vi "countrate_viewer_pix25.vi"() -> ()   [LabVIEW 2022 SP3]
panel:
  in  "Current":u16(ring)=10 items=["010_0417_101816", "020_0417_101556", "040_0417_101120", "060_0417_100851", "080_0417_100615", "100_0417_100344", "120_0417_100115", "140_0417_095846", "160_0417_095605", "180_0417_095308", "200_0417_095036"]
  in  "Path":path=path "C:/Users/User/OneDrive/measurements/pix25/PIX25/17_04_2023/M1/1_CountRate_gate_1s_iKRUM_14_setting_1/TS_step_10"
  in  "Tab Control":enum32{"Single pixel", "Pixels ROI"}(tab)=enum."Pixels ROI"
  out "Counns_vs_Current":cluster{i32[], i32[]}(graph)={[10, 20, 40, 60, 80, 100, 120, 140, 160, 180, 200], [1269, 2399, 4745, 7025, 8884, 10294, 11332, 12142, 12811, 11997, 8843]}
  out "SP_Thscans":i32[][](graph)=[[1, 1, 1, 1, 1, 1, 1, 1, 1, 1, 2, 2, 189750, 27421, 55263, 771071, 189820, 555977, 604477, 176470, 8254, 2553, 2142, 2098, 1983, 1841, 1720, 1662, 1491, 1416, 1364, 1330, 1269, 1152, 1093, 1054, 962, 959, 932, 842, 859, 771, 782, 672, 660, 595, 542, 499, 515, 482, 463, 399, 324, 318, 310, 306, 275, 226, 206, 204, 183, 191, 154, 133, 105, 88, 81, 74, 55, 30, 16, 16, 9, 2, 1, 1, 1, 2, 0, 1, 1, 1, 1, 0, 1, 1, 1, 0, 0, 0, 0, 0, 0, 0, 0, 0, 0, 0, 0, 0, 0], [1, 1, 1, 1, 1, 1, 1, 1, 3, 3, 3, 6, 215655, 123107, 60400, 109023, 562715, 135760, 344132, 161375, 9801, 4778, 4548, 4138, 3957, 3703, 3430, 3172, 3013, 2937, 2749, 2622, 2399, 2350, 2299, 2087, 1990, 1901, 1845, 1667, 1682, 1571, 1407, 1320, 1305, 1218, 1205, 1051, 948, 927, 902, 820, 705, 694, 632, 587, 520, 474, 459, 424, 399, 303, 295, 270, 214, 207, 180, 122, 113, 80, 39, 26, 10, 5, 3, 2, 3, 3, 2, 1, 0, 2, 3, 0, 0, 0, 1, 0, 1, 1, 2, 0, 0, 1, 0, 0, 0, 0, 0, 2, 0], [1, 1, 1, 1, 1, 1, 1, 1, 2, 2, 6, 9, 246177, 154316, 61581, 291268, 92235, 808784, 175375, 162478, 14536, 9814, 8979, 8241, 7781, 7331, 6713, 6502, 6202, 5729, 5414, 5293, 4745, 4666, 4367, 4187, 4099, 3805, 3617, 3379, 3236, 2941, 2924, 2720, 2530, 2322, 2186, 2120, 1914, 1753, 1680, 1555, 1433, 1277, 1214, 1119, 1051, 921, 872, 761, 735, 644, 567, 508, 460, 399, 349, 302, 233, 134, 89, 44, 27, 11, 9, 10, 7, 4, 0, 2, 2, 1, 1, 2, 1, 1, 0, 0, 1, 1, 0, 2, 1, 1, 0, 0, 0, 0, 0, 0, 1], [1, 1, 1, 1, 1, 1, 1, 1, 1, 5, 11, 17, 251777, 562574, 84697, 446485, 689648, 558243, 122437, 148538, 18881, 13957, 12791, 11866, 11229, 10474, 9746, 9238, 8754, 8227, 7810, 7238, 7025, 6523, 6383, 5947, 5555, 5367, 5101, 4876, 4580, 4293, 4092, 3850, 3612, 3351, 3193, 2949, 2792, 2702, 2356, 2236, 2030, 1884, 1737, 1644, 1413, 1411, 1239, 1123, 1113, 932, 832, 746, 629, 568, 503, 412, 288, 228, 116, 62, 33, 22, 14, 6, 9, 5, 7, 4, 4, 3, 2, 5, 1, 2, 2, 1, 3, 1, 1, 0, 0, 1, 0, 0, 1, 0, 0, 0, 0], [1, 1, 1, 1, 1, 1, 1, 1, 2, 7, 9, 9, 202033, 1022635, 119268, 1015096, 454383, 182206, 350774, 170408, 22775, 17422, 15771, 14821, 13787, 12976, 12251, 11478, 10931, 10429, 9679, 9276, 8884, 8347, 7999, 7558, 7315, 6797, 6383, 6210, 5707, 5417, 5063, 4826, 4510, 4230, 3969, 3814, 3585, 3213, 3062, 2900, 2662, 2346, 2209, 1943, 1827, 1688, 1550, 1395, 1307, 1150, 1078, 943, 825, 699, 585, 452, 322, 237, 131, 73, 46, 27, 20, 10, 9, 5, 7, 1, 7, 4, 5, 1, 3, 4, 3, 3, 4, 2, 0, 0, 0, 0, 1, 0, 0, 0, 0, 1, 0], [1, 1, 1, 1, 1, 1, 2, 1, 3, 4, 11, 19, 274433, 736852, 821692, 369364, 339077, 400614, 49867, 156608, 25953, 20145, 18691, 17666, 16423, 15179, 14099, 13351, 12750, 11986, 11698, 10689, 10294, 9752, 9185, 8633, 8319, 7879, 7376, 7210, 6582, 6262, 5932, 5747, 5351, 4921, 4701, 4447, 4104, 3904, 3562, 3318, 3035, 2758, 2556, 2267, 2131, 1940, 1864, 1662, 1461, 1371, 1197, 1084, 930, 806, 719, 580, 439, 277, 172, 95, 36, 26, 14, 12, 12, 10, 8, 10, 4, 1, 5, 7, 5, 2, 2, 1, 5, 1, 2, 1, 0, 1, 2, 0, 1, 0, 0, 0, 1], [1, 1, 1, 1, 1, 1, 1, 2, 4, 7, 10, 12, 311804, 152117, 828999, 642634, 363185, 305129, 867296, 125119, 26655, 22309, 20313, 19079, 17994, 16979, 15927, 14965, 14006, 13378, 12576, 11787, 11332, 10840, 10197, 9767, 9169, 8727, 8266, 7729, 7339, 7013, 6584, 6047, 5921, 5521, 5177, 4875, 4525, 4121, 4020, 3700, 3209, 3060, 2771, 2622, 2360, 2146, 1955, 1821, 1658, 1461, 1314, 1171, 1072, 904, 782, 621, 477, 336, 173, 103, 46, 37, 27, 10, 16, 6, 16, 9, 9, 5, 8, 7, 5, 1, 3, 3, 1, 3, 2, 2, 0, 2, 3, 2, 1, 3, 1, 1, 0], [1, 1, 1, 1, 1, 1, 1, 1, 1, 8, 8, 20, 366384, 586024, 65549, 888105, 959806, 722112, 664736, 126970, 28637, 23922, 22045, 20230, 19190, 18013, 16934, 15760, 15137, 14055, 13485, 12874, 12142, 11633, 10788, 10428, 9923, 9586, 8835, 8358, 7772, 7294, 7183, 6704, 6305, 5917, 5557, 5285, 4911, 4634, 4218, 3980, 3659, 3388, 3186, 2909, 2580, 2378, 2168, 1935, 1806, 1563, 1444, 1285, 1215, 926, 829, 712, 496, 357, 218, 114, 64, 29, 22, 25, 15, 11, 13, 10, 4, 10, 4, 5, 5, 6, 3, 4, 2, 2, 3, 1, 2, 1, 0, 1, 1, 0, 0, 1, 2], [1, 1, 1, 1, 1, 1, 1, 1, 2, 3, 5, 7, 308514, 175649, 361198, 671641, 1026371, 658278, 908428, 135148, 29294, 24322, 22324, 21165, 19477, 18508, 17428, 16326, 15558, 14629, 13820, 13092, 12811, 11864, 11317, 10598, 10203, 9338, 8959, 8586, 8105, 7835, 7134, 6915, 6558, 6290, 5900, 5457, 4961, 4629, 4282, 3990, 3592, 3468, 3141, 2925, 2728, 2386, 2175, 2023, 1855, 1666, 1539, 1284, 1165, 985, 878, 728, 553, 356, 229, 135, 78, 34, 33, 17, 16, 6, 8, 8, 4, 8, 6, 5, 10, 3, 2, 4, 6, 3, 2, 2, 1, 3, 1, 0, 0, 3, 0, 0, 0], [1, 1, 1, 1, 1, 1, 1, 1, 2, 2, 5, 11, 362041, 673975, 623187, 712352, 72767, 287790, 813455, 131860, 28336, 23579, 21491, 20346, 19052, 17661, 16587, 15674, 14749, 14122, 13390, 12559, 11997, 11243, 10817, 10425, 9366, 9242, 8585, 8354, 7747, 7409, 7150, 6494, 6059, 5904, 5530, 5039, 4786, 4402, 4174, 3906, 3672, 3341, 3065, 2840, 2530, 2366, 2156, 1953, 1762, 1622, 1492, 1271, 1165, 972, 858, 703, 510, 331, 214, 148, 69, 47, 22, 30, 15, 11, 12, 13, 10, 15, 6, 12, 5, 7, 1, 3, 4, 4, 1, 2, 1, 1, 3, 0, 0, 1, 0, 0, 0], [1, 1, 1, 1, 1, 1, 1, 1, 1, 2, 2, 9, 291425, 195362, 891949, 260720, 603938, 253434, 410135, 175520, 23257, 17183, 16078, 14754, 13718, 12922, 12197, 11578, 11092, 10303, 9717, 9350, 8843, 8441, 7803, 7662, 7122, 6707, 6354, 6082, 5631, 5399, 5193, 4886, 4424, 4377, 4047, 3830, 3535, 3386, 3095, 3018, 2727, 2562, 2307, 2125, 1961, 1757, 1703, 1477, 1338, 1287, 1168, 1072, 906, 794, 641, 532, 392, 294, 183, 101, 93, 49, 25, 24, 16, 15, 8, 13, 15, 11, 5, 12, 3, 4, 4, 6, 4, 3, 4, 1, 0, 1, 2, 3, 1, 1, 0, 1, 0]]
  out "ROI_Thscans":i32[][](graph)
  out "ROI Counns_vs_Current":cluster{"x":i32[], "y":i32[]}[](graph)=[{"x"=[10, 20, 40, 60, 80, 100, 120, 140, 160, 180, 200], "y"=[5788, 11550, 22908, 34725, 46596, 58476, 69984, 80642, 89685, 96090, 95086]}, {"x"=[10, 20, 40, 60, 80, 100, 120, 140, 160, 180, 200], "y"=[5229, 10481, 21003, 31934, 43040, 53953, 63920, 73197, 81464, 86557, 82444]}, {"x"=[10, 20, 40, 60, 80, 100, 120, 140, 160, 180, 200], "y"=[6347, 12619, 24813, 37516, 50152, 62999, 76048, 88087, 97906, 105623, 107728]}, {"x"=[10, 20, 40, 60, 80, 100, 120, 140, 160, 180, 200], "y"=[5885, 12506, 24598, 33614, 44225, 60163, 71358, 71080, 88038, 99015, 103830]}, {"x"=[10, 20, 40, 60, 80, 100, 120, 140, 160, 180, 200], "y"=[7259, 14155, 27794, 42464, 55513, 68152, 83308, 97868, 111207, 117116, 122425]}, {"x"=[10, 20, 40, 60, 80, 100, 120, 140, 160, 180, 200], "y"=[6068, 11921, 24401, 36511, 48958, 61586, 73018, 85686, 98316, 100964, 106641]}, {"x"=[10, 20, 40, 60, 80, 100, 120, 140, 160, 180, 200], "y"=[5792, 11917, 25031, 37218, 50888, 63603, 76543, 90713, 98707, 107263, 103432]}, {"x"=[10, 20, 40, 60, 80, 100, 120, 140, 160, 180, 200], "y"=[5642, 11098, 21720, 33554, 45976, 58183, 67268, 77320, 84854, 93133, 85305]}, {"x"=[10, 20, 40, 60, 80, 100, 120, 140, 160, 180, 200], "y"=[4783, 9367, 19364, 30110, 40670, 52250, 61461, 68636, 71992, 73708, 66528]}, {"x"=[10, 20, 40, 60, 80, 100, 120, 140, 160, 180, 200], "y"=[6141, 12215, 23243, 35325, 46885, 54262, 66265, 74464, 84272, 95326, 103957]}, {"x"=[10, 20, 40, 60, 80, 100, 120, 140, 160, 180, 200], "y"=[6203, 12445, 23795, 36401, 47597, 60300, 71348, 83522, 92454, 105103, 105201]}, {"x"=[10, 20, 40, 60, 80, 100, 120, 140, 160, 180, 200], "y"=[6409, 12362, 24510, 36727, 48593, 60932, 73260, 84142, 99493, 104084, 102507]}, {"x"=[10, 20, 40, 60, 80, 100, 120, 140, 160, 180, 200], "y"=[5600, 10780, 21268, 32773, 44254, 56029, 68450, 78702, 89054, 95249, 91650]}, {"x"=[10, 20, 40, 60, 80, 100, 120, 140, 160, 180, 200], "y"=[5730, 11768, 23959, 37583, 51069, 65900, 77496, 87689, 90185, 88684, 82954]}, {"x"=[10, 20, 40, 60, 80, 100, 120, 140, 160, 180, 200], "y"=[4950, 9918, 20223, 31416, 43335, 51753, 63319, 71716, 76073, 80119, 73536]}, {"x"=[10, 20, 40, 60, 80, 100, 120, 140, 160, 180, 200], "y"=[5855, 11461, 22694, 33519, 44291, 54105, 63924, 75411, 84569, 90629, 94843]}, {"x"=[10, 20, 40, 60, 80, 100, 120, 140, 160, 180, 200], "y"=[7035, 13784, 26383, 39929, 53572, 64999, 77282, 92097, 103221, 112618, 117835]}, {"x"=[10, 20, 40, 60, 80, 100, 120, 140, 160, 180, 200], "y"=[5765, 11431, 22765, 34091, 46220, 56797, 69511, 81444, 89921, 98431, 97594]}, {"x"=[10, 20, 40, 60, 80, 100, 120, 140, 160, 180, 200], "y"=[5960, 11917, 23994, 36280, 49990, 62024, 74217, 91174, 99338, 105110, 100869]}, {"x"=[10, 20, 40, 60, 80, 100, 120, 140, 160, 180, 200], "y"=[5270, 10448, 20294, 32674, 44417, 56893, 68709, 77593, 86101, 90185, 82577]}, {"x"=[10, 20, 40, 60, 80, 100, 120, 140, 160, 180, 200], "y"=[5359, 10654, 22577, 35638, 47792, 61620, 74326, 84194, 92202, 95489, 86340]}, {"x"=[10, 20, 40, 60, 80, 100, 120, 140, 160, 180, 200], "y"=[6457, 12820, 25205, 37866, 48731, 60735, 70570, 80672, 88335, 98136, 114030]}, {"x"=[10, 20, 40, 60, 80, 100, 120, 140, 160, 180, 200], "y"=[5797, 11642, 22214, 32620, 43952, 52970, 65365, 76095, 85027, 94971, 99189]}, {"x"=[10, 20, 40, 60, 80, 100, 120, 140, 160, 180, 200], "y"=[6493, 13283, 25578, 38607, 51756, 65289, 78759, 90712, 102590, 112174, 113346]}, {"x"=[10, 20, 40, 60, 80, 100, 120, 140, 160, 180, 200], "y"=[6131, 12307, 23551, 36815, 47661, 62888, 75943, 87844, 97315, 101982, 101180]}, {"x"=[10, 20, 40, 60, 80, 100, 120, 140, 160, 180, 200], "y"=[5259, 10834, 21749, 33639, 45440, 57438, 67358, 78134, 85389, 90884, 82024]}, {"x"=[10, 20, 40, 60, 80, 100, 120, 140, 160, 180, 200], "y"=[5026, 10318, 21215, 32005, 44148, 54883, 64405, 72077, 78718, 81244, 72589]}, {"x"=[10, 20, 40, 60, 80, 100, 120, 140, 160, 180, 200], "y"=[5582, 11514, 22061, 33105, 43254, 53653, 62929, 72403, 81026, 90626, 100266]}, {"x"=[10, 20, 40, 60, 80, 100, 120, 140, 160, 180, 200], "y"=[6515, 13112, 25125, 38215, 50598, 59696, 72448, 86988, 92126, 106792, 112252]}, {"x"=[10, 20, 40, 60, 80, 100, 120, 140, 160, 180, 200], "y"=[5871, 11473, 22330, 34446, 46442, 59285, 70761, 83949, 95121, 101300, 100708]}, {"x"=[10, 20, 40, 60, 80, 100, 120, 140, 160, 180, 200], "y"=[5975, 11687, 23489, 38233, 51732, 64832, 78464, 90732, 100917, 108118, 99798]}, {"x"=[10, 20, 40, 60, 80, 100, 120, 140, 160, 180, 200], "y"=[6661, 13099, 26413, 39649, 53440, 67206, 82751, 93695, 99245, 104438, 102789]}, {"x"=[10, 20, 40, 60, 80, 100, 120, 140, 160, 180, 200], "y"=[4751, 9818, 20106, 31147, 42094, 53245, 62450, 70843, 77155, 77204, 68750]}, {"x"=[10, 20, 40, 60, 80, 100, 120, 140, 160, 180, 200], "y"=[5815, 11487, 23408, 33532, 43607, 53632, 62532, 72778, 91492, 87705, 93606]}, {"x"=[10, 20, 40, 60, 80, 100, 120, 140, 160, 180, 200], "y"=[6145, 12137, 24283, 35912, 47984, 60042, 71197, 82450, 91465, 101640, 106800]}, {"x"=[10, 20, 40, 60, 80, 100, 120, 140, 160, 180, 200], "y"=[5839, 12102, 23689, 34731, 47713, 58801, 72762, 84188, 95085, 103475, 101085]}, {"x"=[10, 20, 40, 60, 80, 100, 120, 140, 160, 180, 200], "y"=[6521, 13603, 26423, 40081, 53619, 67033, 81659, 94386, 102889, 112719, 101456]}, {"x"=[10, 20, 40, 60, 80, 100, 120, 140, 160, 180, 200], "y"=[5739, 11197, 23126, 35612, 47982, 62907, 73736, 83529, 91879, 97873, 91141]}, {"x"=[10, 20, 40, 60, 80, 100, 120, 140, 160, 180, 200], "y"=[4776, 10027, 20606, 32724, 45375, 55568, 68749, 77146, 85954, 87124, 78963]}, {"x"=[10, 20, 40, 60, 80, 100, 120, 140, 160, 180, 200], "y"=[6465, 12945, 25114, 37590, 48827, 59668, 70517, 82063, 86884, 102328, 112073]}, {"x"=[10, 20, 40, 60, 80, 100, 120, 140, 160, 180, 200], "y"=[6207, 12819, 24802, 36733, 48964, 60019, 73296, 82568, 95584, 103564, 111240]}, {"x"=[10, 20, 40, 60, 80, 100, 120, 140, 160, 180, 200], "y"=[6078, 11835, 23313, 35613, 48090, 59502, 70746, 83346, 92527, 100503, 98288]}, {"x"=[10, 20, 40, 60, 80, 100, 120, 140, 160, 180, 200], "y"=[6193, 12155, 24087, 37497, 49914, 62886, 79012, 89470, 101446, 105122, 106578]}, {"x"=[10, 20, 40, 60, 80, 100, 120, 140, 160, 180, 200], "y"=[5811, 11991, 23388, 36058, 48982, 61667, 73617, 84283, 93739, 96720, 89162]}, {"x"=[10, 20, 40, 60, 80, 100, 120, 140, 160, 180, 200], "y"=[4886, 9903, 19341, 30333, 40315, 52926, 62987, 71919, 76575, 80727, 72620]}, {"x"=[10, 20, 40, 60, 80, 100, 120, 140, 160, 180, 200], "y"=[5917, 11703, 22607, 32632, 44146, 54678, 61541, 69228, 77442, 83939, 88770]}, {"x"=[10, 20, 40, 60, 80, 100, 120, 140, 160, 180, 200], "y"=[6360, 12712, 25071, 37607, 49119, 61550, 73999, 87091, 99370, 110387, 117315]}, {"x"=[10, 20, 40, 60, 80, 100, 120, 140, 160, 180, 200], "y"=[5637, 10800, 21419, 31264, 42918, 52823, 63600, 74037, 85304, 92844, 92865]}, {"x"=[10, 20, 40, 60, 80, 100, 120, 140, 160, 180, 200], "y"=[6220, 12356, 24573, 37282, 46557, 62650, 77112, 90296, 96570, 105338, 98824]}, {"x"=[10, 20, 40, 60, 80, 100, 120, 140, 160, 180, 200], "y"=[5946, 11720, 22796, 34835, 47576, 61628, 74813, 81560, 88298, 94278, 89055]}, {"x"=[10, 20, 40, 60, 80, 100, 120, 140, 160, 180, 200], "y"=[4651, 9451, 20681, 30069, 45212, 52739, 60191, 77864, 84655, 86936, 76579]}, {"x"=[10, 20, 40, 60, 80, 100, 120, 140, 160, 180, 200], "y"=[5889, 11281, 22190, 31896, 40719, 51446, 59490, 68869, 78595, 86368, 91330]}, {"x"=[10, 20, 40, 60, 80, 100, 120, 140, 160, 180, 200], "y"=[6630, 12783, 24842, 37375, 48062, 59641, 71324, 81593, 90246, 97990, 104775]}, {"x"=[10, 20, 40, 60, 80, 100, 120, 140, 160, 180, 200], "y"=[5867, 11588, 22851, 33832, 47580, 60283, 70110, 82428, 96106, 103789, 98846]}, {"x"=[10, 20, 40, 60, 80, 100, 120, 140, 160, 180, 200], "y"=[6433, 13032, 25341, 39210, 52431, 65238, 82194, 94816, 104057, 110054, 109354]}, {"x"=[10, 20, 40, 60, 80, 100, 120, 140, 160, 180, 200], "y"=[4915, 9914, 21494, 33076, 44294, 56920, 67429, 73270, 86682, 91358, 86386]}, {"x"=[10, 20, 40, 60, 80, 100, 120, 140, 160, 180, 200], "y"=[4611, 9128, 18396, 29533, 42824, 55432, 65914, 75697, 77030, 74034, 65796]}, {"x"=[10, 20, 40, 60, 80, 100, 120, 140, 160, 180, 200], "y"=[6137, 12103, 24402, 35787, 46322, 56926, 68189, 78092, 88057, 96498, 103136]}, {"x"=[10, 20, 40, 60, 80, 100, 120, 140, 160, 180, 200], "y"=[5341, 10444, 20124, 29946, 40031, 49103, 59705, 69520, 78755, 87109, 92424]}, {"x"=[10, 20, 40, 60, 80, 100, 120, 140, 160, 180, 200], "y"=[6347, 12678, 25005, 37948, 50926, 63899, 77741, 91027, 102143, 113237, 111110]}, {"x"=[10, 20, 40, 60, 80, 100, 120, 140, 160, 180, 200], "y"=[5896, 11568, 23123, 35248, 47989, 60353, 71932, 85292, 93325, 98051, 96866]}, {"x"=[10, 20, 40, 60, 80, 100, 120, 140, 160, 180, 200], "y"=[5621, 11047, 21641, 34136, 46265, 58159, 71885, 81485, 90722, 94160, 87324]}, {"x"=[10, 20, 40, 60, 80, 100, 120, 140, 160, 180, 200], "y"=[4908, 10240, 20741, 31984, 42422, 54864, 64949, 74232, 78588, 79502, 74459]}, {"x"=[10, 20, 40, 60, 80, 100, 120, 140, 160, 180, 200], "y"=[5519, 11315, 22027, 32503, 44054, 53734, 63339, 68779, 79605, 90438, 94246]}, {"x"=[10, 20, 40, 60, 80, 100, 120, 140, 160, 180, 200], "y"=[5327, 10564, 20408, 30522, 40634, 50688, 60780, 70850, 82725, 89584, 94259]}, {"x"=[10, 20, 40, 60, 80, 100, 120, 140, 160, 180, 200], "y"=[5187, 10424, 20525, 31012, 41198, 52463, 61740, 72292, 80737, 88660, 92462]}, {"x"=[10, 20, 40, 60, 80, 100, 120, 140, 160, 180, 200], "y"=[6370, 12815, 25194, 38037, 52694, 66015, 80638, 94768, 104818, 109896, 103806]}, {"x"=[10, 20, 40, 60, 80, 100, 120, 140, 160, 180, 200], "y"=[5723, 10990, 22726, 34728, 45870, 62613, 72672, 81240, 94012, 98624, 94279]}, {"x"=[10, 20, 40, 60, 80, 100, 120, 140, 160, 180, 200], "y"=[5559, 11192, 22678, 35288, 48484, 61341, 72279, 82473, 89803, 91719, 83563]}, {"x"=[10, 20, 40, 60, 80, 100, 120, 140, 160, 180, 200], "y"=[6005, 12042, 23062, 34393, 44232, 53695, 63943, 74377, 83983, 92363, 99282]}, {"x"=[10, 20, 40, 60, 80, 100, 120, 140, 160, 180, 200], "y"=[5794, 11547, 22710, 33545, 44618, 55489, 66517, 76634, 86503, 95392, 101789]}, {"x"=[10, 20, 40, 60, 80, 100, 120, 140, 160, 180, 200], "y"=[5837, 11660, 22902, 33966, 46069, 58176, 70161, 82035, 93023, 101031, 102975]}, {"x"=[10, 20, 40, 60, 80, 100, 120, 140, 160, 180, 200], "y"=[6053, 11435, 23633, 35910, 47721, 60268, 72564, 83037, 92895, 99531, 95991]}, {"x"=[10, 20, 40, 60, 80, 100, 120, 140, 160, 180, 200], "y"=[6258, 12469, 24752, 38229, 51998, 64560, 79473, 91376, 97613, 104591, 96109]}, {"x"=[10, 20, 40, 60, 80, 100, 120, 140, 160, 180, 200], "y"=[4745, 9591, 19882, 31415, 42795, 54495, 64641, 72414, 77929, 80465, 74201]}, {"x"=[10, 20, 40, 60, 80, 100, 120, 140, 160, 180, 200], "y"=[5890, 11920, 23303, 34657, 45365, 55920, 65499, 75196, 82071, 93600, 101374]}, {"x"=[10, 20, 40, 60, 80, 100, 120, 140, 160, 180, 200], "y"=[6541, 12794, 25171, 36938, 48706, 60632, 71441, 88076, 93485, 103440, 108524]}, {"x"=[10, 20, 40, 60, 80, 100, 120, 140, 160, 180, 200], "y"=[5655, 11337, 22572, 34920, 46195, 57303, 68226, 77536, 91103, 95817, 102231]}, {"x"=[10, 20, 40, 60, 80, 100, 120, 140, 160, 180, 200], "y"=[6626, 13255, 26320, 40370, 54265, 67717, 82949, 96862, 107169, 113581, 108973]}, {"x"=[10, 20, 40, 60, 80, 100, 120, 140, 160, 180, 200], "y"=[5007, 10140, 19755, 29852, 40078, 51879, 61423, 71617, 79569, 84995, 75201]}, {"x"=[10, 20, 40, 60, 80, 100, 120, 140, 160, 180, 200], "y"=[5334, 10982, 21744, 34144, 47626, 59909, 72436, 82566, 84666, 86131, 77781]}, {"x"=[10, 20, 40, 60, 80, 100, 120, 140, 160, 180, 200], "y"=[6084, 12087, 23285, 34517, 44678, 55291, 64703, 74419, 83810, 94472, 100272]}, {"x"=[10, 20, 40, 60, 80, 100, 120, 140, 160, 180, 200], "y"=[5164, 10216, 19707, 29678, 38834, 48652, 58129, 66631, 75838, 84002, 91042]}, {"x"=[10, 20, 40, 60, 80, 100, 120, 140, 160, 180, 200], "y"=[5820, 11498, 22338, 33675, 45330, 56861, 67623, 79589, 87076, 93086, 95194]}, {"x"=[10, 20, 40, 60, 80, 100, 120, 140, 160, 180, 200], "y"=[5774, 11404, 23271, 36059, 47887, 61395, 73184, 84913, 95896, 103925, 99419]}, {"x"=[10, 20, 40, 60, 80, 100, 120, 140, 160, 180, 200], "y"=[5888, 11334, 22798, 34962, 47261, 60599, 72413, 82649, 93459, 96465, 87559]}, {"x"=[10, 20, 40, 60, 80, 100, 120, 140, 160, 180, 200], "y"=[5001, 10473, 21191, 32918, 45508, 57752, 67568, 75288, 84375, 85714, 80045]}, {"x"=[10, 20, 40, 60, 80, 100, 120, 140, 160, 180, 200], "y"=[5980, 11777, 23028, 34868, 46002, 56858, 65963, 76769, 85511, 94476, 103688]}, {"x"=[10, 20, 40, 60, 80, 100, 120, 140, 160, 180, 200], "y"=[6195, 12294, 23971, 34973, 46585, 58801, 69267, 80044, 91049, 100823, 105158]}, {"x"=[10, 20, 40, 60, 80, 100, 120, 140, 160, 180, 200], "y"=[5630, 11163, 21926, 32709, 43989, 55769, 66330, 76422, 88035, 95997, 94069]}, {"x"=[10, 20, 40, 60, 80, 100, 120, 140, 160, 180, 200], "y"=[5857, 11599, 23570, 35384, 47865, 60303, 74962, 84949, 94807, 101965, 103666]}, {"x"=[10, 20, 40, 60, 80, 100, 120, 140, 160, 180, 200], "y"=[5007, 10073, 19834, 30441, 41982, 52912, 63872, 74633, 81127, 84755, 79298]}, {"x"=[10, 20, 40, 60, 80, 100, 120, 140, 160, 180, 200], "y"=[5078, 10291, 20946, 32363, 44816, 56083, 67671, 77244, 84536, 87080, 68102]}]
  out "Image":i32[][](graph)
  in  "ThScan_Load":bool
  in  "Exit":bool
  # "counts vs. current for single pixel for single vt"
  # "thscans of all currents for single pixel"
  # "counts vs. current for ROI pixels for single vt"
  # "thscans of ROI pixels for single current"
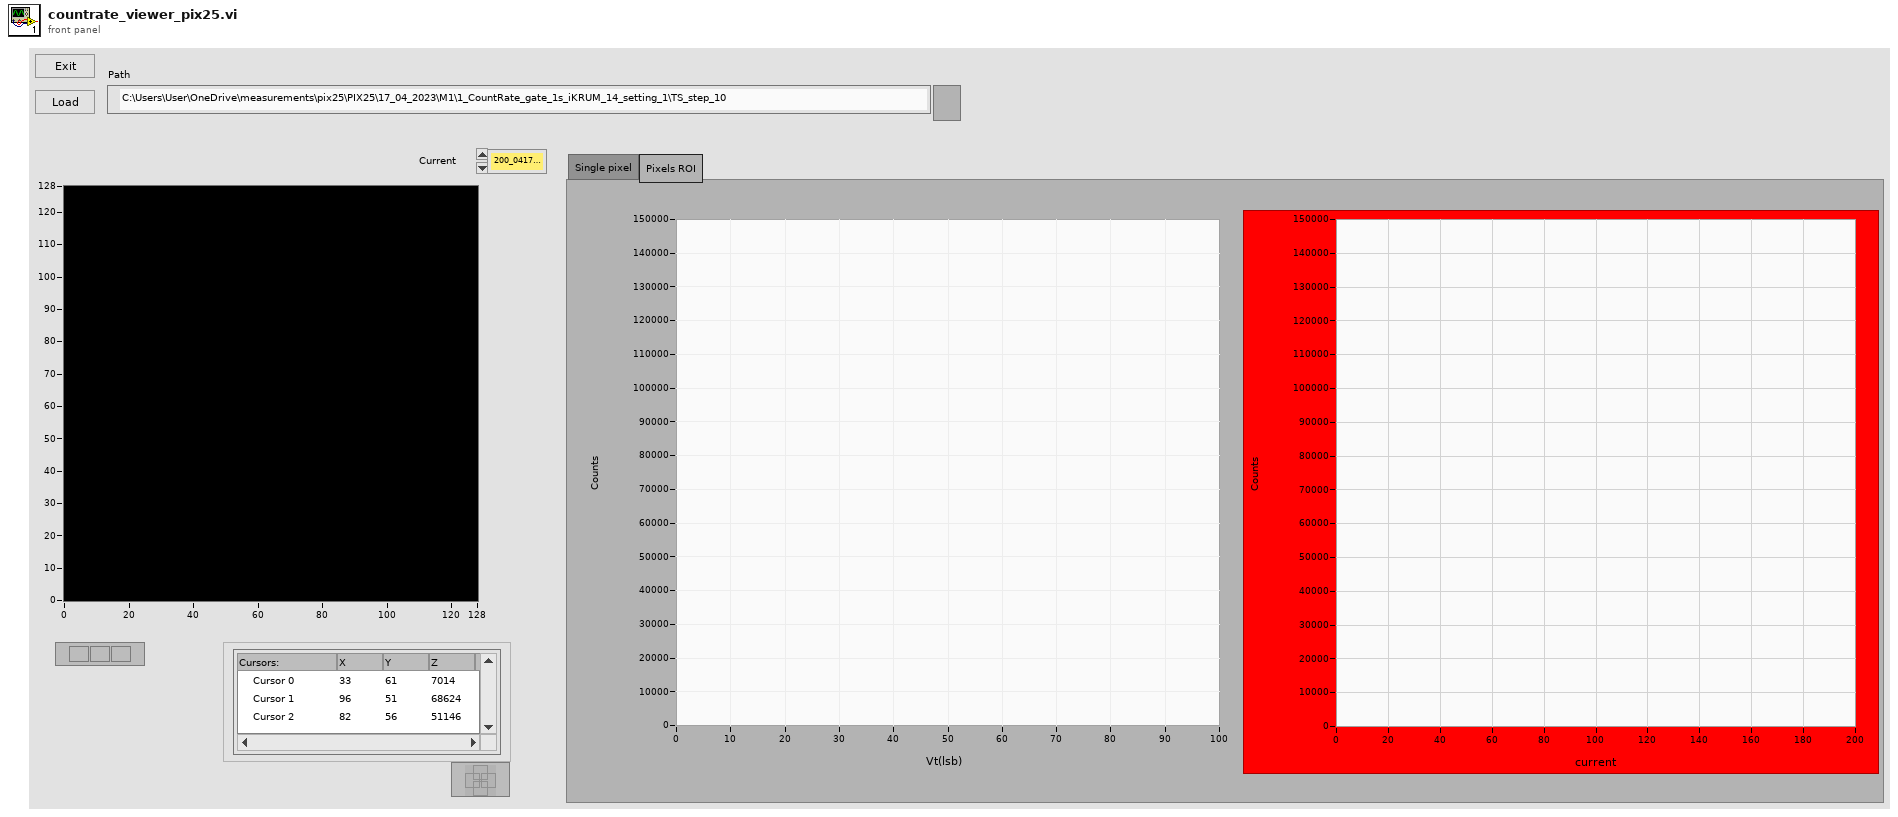
[diagram p1: front panel]
types:
  T1 = typedef "LVPointDoubleTypeDef.ctl" = cluster{"Cursor X":dbl, "Cursor Y":dbl}
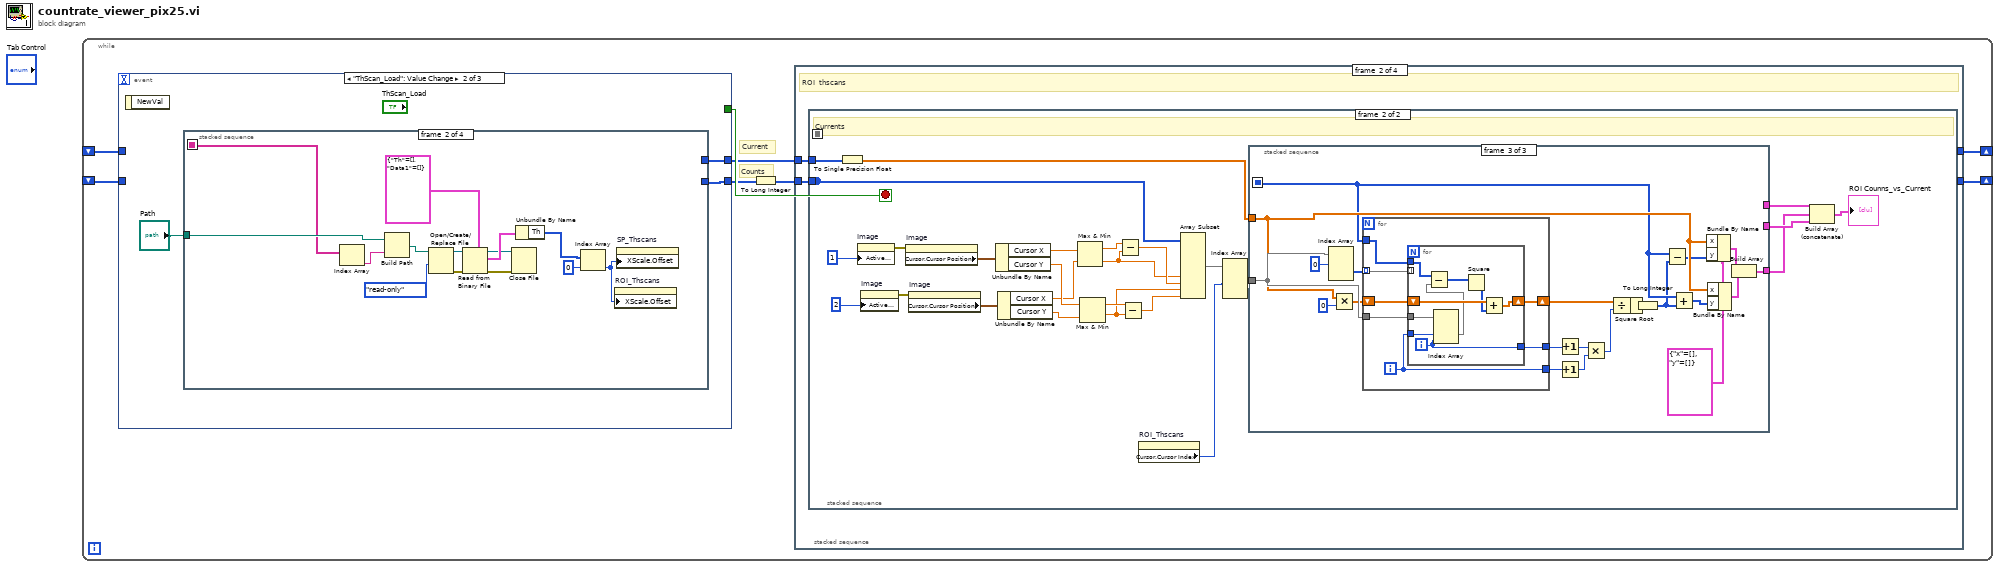
[diagram p0: block diagram]
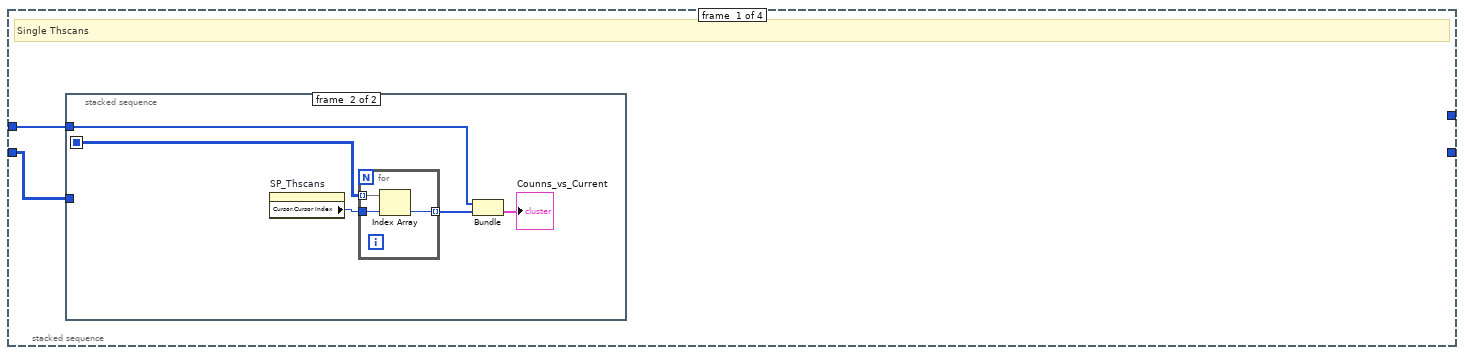
[diagram p2: hidden frame]
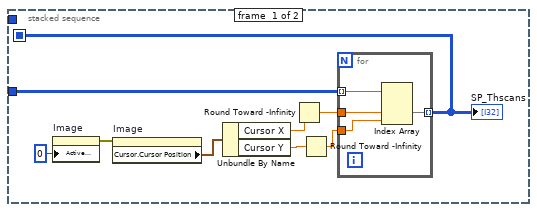
[diagram p3: hidden frame]
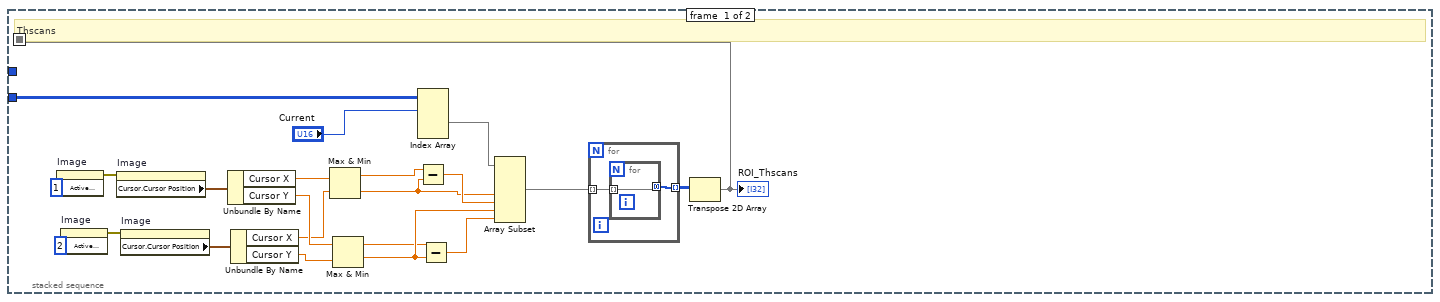
[diagram p4: hidden frame]
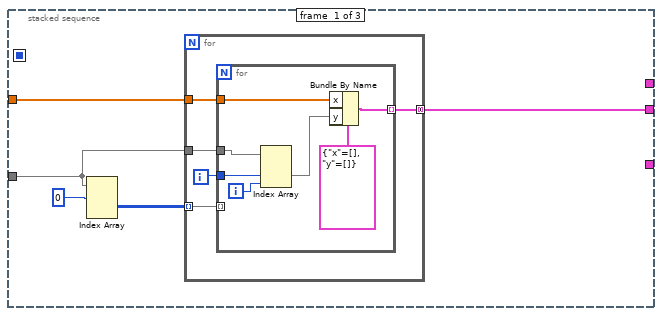
[diagram p5: hidden frame]
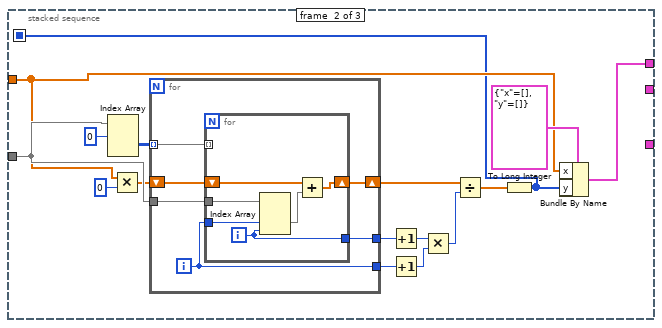
[diagram p6: hidden frame]
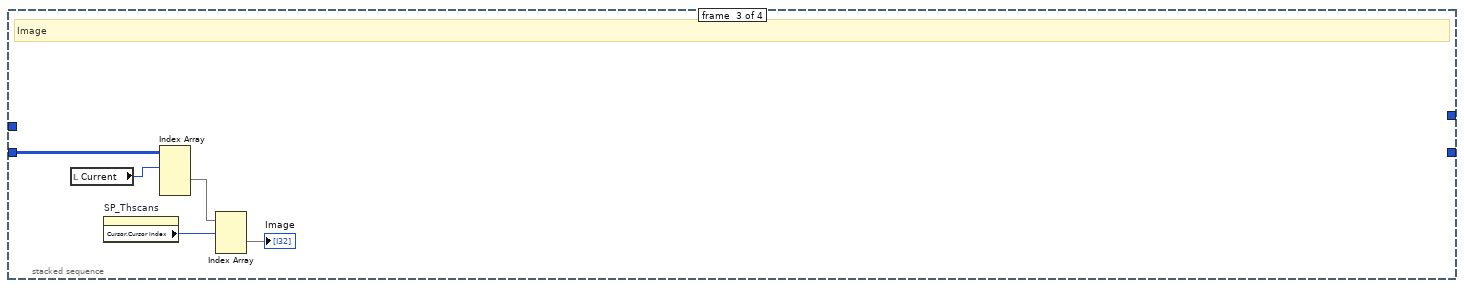
[diagram p7: hidden frame]
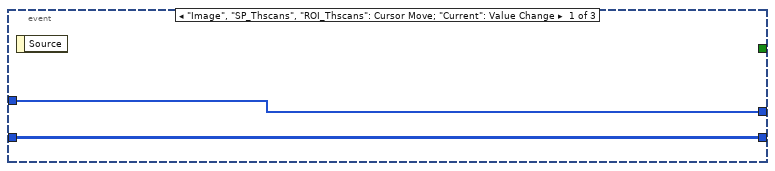
[diagram p9: hidden frame]
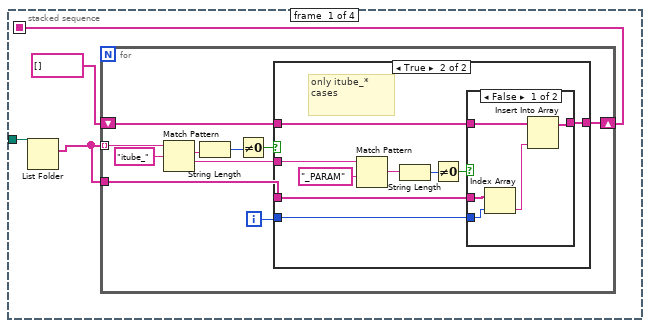
[diagram p10: hidden frame]
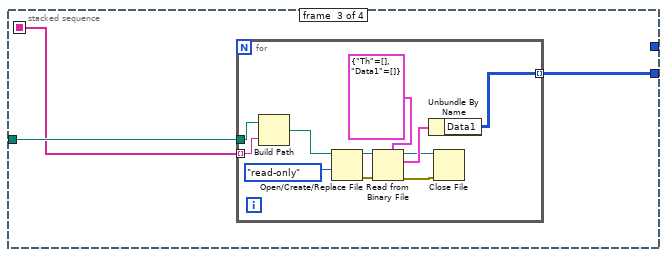
[diagram p13: hidden frame]
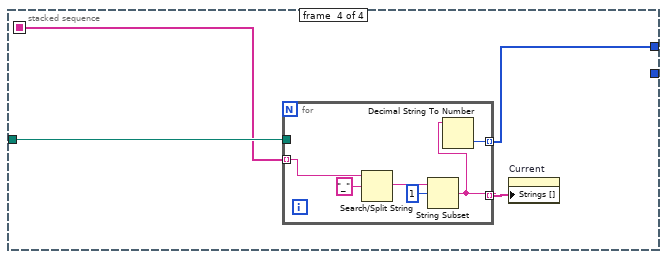
[diagram p14: hidden frame]
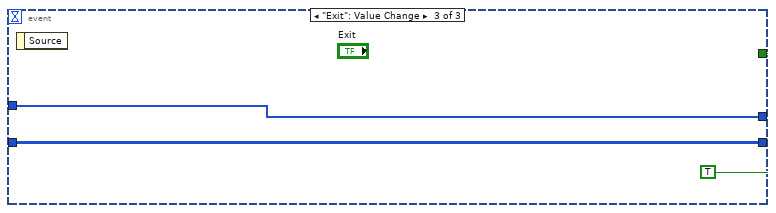
[diagram p15: hidden frame]
diagram:
  n1 = while {
    shift-right: [w5] -> _
    shift-left: _ -> [w7]
    shift-right: [w2] -> _
    shift-left: _ -> [w4]
    stop <- w8 stop-if-true
    # "Counts"
    # "Current"
    n2 = event shown="[1] \"ThScan_Load\": Value Change" {
      selector: _ -> [_ _ _]
      dyn-events: _ -> [_ _ _]
      timeout: _ -> [_ _ _]
      tunnel: [_ _ TRUE] -> w8
      tunnel: w7 -> [w176 _ w249]
      tunnel: [w176 w179 w249] -> w6
      tunnel: w4 -> [w175 _ w248]
      tunnel: [w175 w178 w248] -> w3
      event "Image", "SP_Thscans", "ROI_Thscans": Cursor Move; "Current": Value Change {
        n3 = event-data() -> ()  [unwired: 1 in, 1 out]
      }
      event "ThScan_Load": Value Change {
        n4 = event-data() -> ()  [unwired: 1 in, 1 out]
        n5 = stacked-sequence {
          seq-local: [w180 _ _ _] -> [_ w210 w224 w238]
          tunnel: [_ _ w226 _] -> w179
          tunnel: "Path" -> [w181 w213 w225 w240]
          tunnel: [_ _ _ w239] -> w178
          frame #0 {
            n6 = List Folder(path=w181) -> (filenames=w183:string[])  [unwired: 3 in, 3 out]
            n7 = for {
              tunnel: w183 -> [w193] mode=indexing
              shift-right: [w189] -> w180
              shift-left: string[] [] ("filenames") -> [w190]
              tunnel: w183 -> [w184]
              i -> [w188]
              n8 = Match Pattern(string=w193, regular expression="itube_") -> (match substring=w187:string, after substring=w191:string)  [unwired: 1 in, 2 out]
              n9 = String Length(string=w187) -> (length=w186:i32)
              n10 = Not Equal To 0?(x=w186) -> (x != 0?=w185:bool)
              n11 = case shown="True" w185 {
                tunnel: w191 -> [_ w195]
                tunnel: w190 -> [w194 w199]
                tunnel: [w194 w198] -> w189
                tunnel: w188 -> [_ w197]
                tunnel: w184 -> [_ w196]
                frame False {
                }
                frame True {
                  # "only itube_*\ncases"
                  n12 = Match Pattern(string=w195, regular expression="_PARAM") -> (match substring=w202:string)  [unwired: 1 in, 3 out]
                  n13 = String Length(string=w202) -> (length=w201:i32)
                  n14 = Not Equal To 0?(x=w201) -> (x != 0?=w200:bool)
                  n15 = case shown="False" w200 {
                    tunnel: w199 -> [w207 w209]
                    tunnel: [w204 w209] -> w198
                    tunnel: w197 -> [w206 _]
                    tunnel: w196 -> [w208 _]
                    frame False {
                      n16 = Index Array(array=w208, index=w206) -> (element=w205:string)
                      n17 = Insert Into Array(array=w207, new element=w205) -> (w204:string[])  [unwired: 1 in]
                    }
                    frame True {
                    }
                  }
                }
              }
            }
          }
          frame #1 {
            n18 = Index Array(array=w210) -> (element=w212:string)  [unwired: 1 in]
            n19 = Build Path(base path=w213, name or relative path=w212) -> (appended path=w211:path)
            n20 = Open/Create/Replace File(file path (use dialog)=w211, access (0:read/write)=enum16{"read/write", "read-only", "write-only"}."read-only") -> (refnum out=w220:refnum<file>, error out=w219:errorcluster)  [unwired: 4 in, 1 out]
            n21 = Read from Binary File(5:cluster{"Th":u16[], "Data1":u32[][][]} {"Th"=[], "Data1"=[]} ("TH Gate Scan"), 8:w219, 11:w220) -> (0:w222:errorcluster, 2:w223:cluster{"Th":u16[], "Data1":u32[][][]}, 3:w221:refnum<file>)  [unwired: 3 in, 1 out]
            n22 = Close File(refnum=w221, error in=w222) -> ()  [unwired: 2 out]
            n23 = Unbundle By Name(w223) -> ("Th"=w214:u16[])
            n24 = Index Array(array=w214, index=0) -> (element=w215:u16)
            n25 = property on="ROI_Thscans" class="WFGraph (strict)"("XScale.Offset"=w215) -> ()  [unwired: 2 in, 2 out]
            n26 = property on="SP_Thscans" class="WFGraph (strict)"("XScale.Offset"=w215) -> ()  [unwired: 2 in, 2 out]
          }
          frame #2 {
            n27 = for {
              tunnel: [w230] -> w226 mode=indexing
              tunnel: w224 -> [w228] mode=indexing
              tunnel: w225 -> [w229]
              n28 = Build Path(base path=w229, name or relative path=w228) -> (appended path=w227:path)
              n29 = Open/Create/Replace File(file path (use dialog)=w227, access (0:read/write)=enum16{"read/write", "read-only", "write-only"}."read-only") -> (refnum out=w234:refnum<file>, error out=w233:errorcluster)  [unwired: 4 in, 1 out]
              n30 = Read from Binary File(5:cluster{"Th":u16[], "Data1":u32[][][]} {"Th"=[], "Data1"=[]} ("TH Gate Scan"), 8:w233, 11:w234) -> (0:w236:errorcluster, 2:w237:cluster{"Th":u16[], "Data1":u32[][][]}, 3:w235:refnum<file>)  [unwired: 3 in, 1 out]
              n31 = Unbundle By Name(w237) -> ("Data1"=w230:u32[][][])
              n32 = Close File(refnum=w235, error in=w236) -> ()  [unwired: 2 out]
            }
          }
          frame #3 {
            n33 = for {
              tunnel: w238 -> [w244] mode=indexing
              tunnel: [w243] -> w241 mode=indexing
              tunnel: w240 -> [_]
              tunnel: [w242] -> w239 mode=indexing
              n34 = Search/Split String(string=w244, search string/char (-)="_") -> (match + rest of string=w246:string)  [unwired: 1 in, 2 out]
              n35 = String Subset(string=w246, offset (0)=1) -> (substring=w243:string)  [unwired: 1 in]
              n36 = Decimal String To Number(string=w243) -> (number=w242:i32)  [unwired: 2 in, 1 out]
            }
            n37 = property on="Current" class="Ring (strict)"("Strings []"=w241) -> ()  [unwired: 2 in, 2 out]
          }
        }
      }
      event "Exit": Value Change {
        n38 = event-data() -> ()  [unwired: 1 in, 1 out]
      }
    }
    n39 = To Long Integer(number=w6) -> (32bit integer=w1:i32[][][][])
    n40 = stacked-sequence {
      tunnel: w1 -> [w10 w33 w168 w174]
      tunnel: [_ _ _ w174] -> w5
      tunnel: w3 -> [w9 w32 _ w173]
      tunnel: [_ _ _ w173] -> w2
      tunnel: [_ w33 _ _] -> _
      frame #0 {
        # "Single Thscans"
        n41 = stacked-sequence {
          seq-local: [w11 _] -> [_ w24]
          tunnel: w10 -> [w12 _]
          tunnel: w9 -> [_ w25]
          frame #0 {
            n42 = property on="Image" class="IntGraph (strict)"("Active Cursor"=u32 0) -> (error out=w14:errorcluster)  [unwired: 2 in, 1 out]
            n43 = property on="Image" class="IntGraph (strict)"(error in=w14) -> ("Cursor.Cursor Position"=w15:T1)  [unwired: 1 in, 2 out]
            n44 = Unbundle By Name(w15) -> ("Cursor X"=w17:dbl, "Cursor Y"=w18:dbl)
            n45 = Round Toward -Infinity(1:w17) -> (0:w16:dbl)
            n46 = Round Toward -Infinity(1:w18) -> (0:w19:dbl)
            n47 = for {
              tunnel: w19 -> [w23]
              tunnel: w16 -> [w22]
              tunnel: w12 -> [w21] mode=indexing
              tunnel: [w20] -> w11 mode=indexing
              n48 = Index Array(array=w21, index (dim 1)=w22, index (dim 2)=w23) -> (element=w20:i32[])  [unwired: 1 in]
            }
            "SP_Thscans" <- w11
          }
          frame #1 {
            n49 = property on="SP_Thscans" class="WFGraph (strict)"() -> ("Cursor.Cursor Index"=w26:i32)  [unwired: 2 in, 2 out]
            n50 = for {
              tunnel: w24 -> [w31] mode=indexing
              tunnel: w26 -> [w30]
              tunnel: [w29] -> w27 mode=indexing
              n51 = Index Array(array=w31, index=w30) -> (element=w29:i32)
            }
            n52 = Bundle(w25, w27) -> (→"Counns_vs_Current":cluster{i32[], i32[]})  [unwired: 1 in]
          }
        }
      }
      frame #1 {
        # "ROI  thscans"
        n53 = stacked-sequence {
          seq-local: [w34 _] -> [_ _]
          tunnel: w33 -> [w35 w72]
          tunnel: w32 -> [_ w65]
          frame #0 {
            # "Thscans"
            n54 = property on="Image" class="IntGraph (strict)"("Active Cursor"=u32 1) -> (error out=w42:errorcluster)  [unwired: 2 in, 1 out]
            n55 = property on="Image" class="IntGraph (strict)"("Active Cursor"=u32 2) -> (error out=w43:errorcluster)  [unwired: 2 in, 1 out]
            n56 = property on="Image" class="IntGraph (strict)"(error in=w42) -> ("Cursor.Cursor Position"=w44:T1)  [unwired: 1 in, 2 out]
            n57 = property on="Image" class="IntGraph (strict)"(error in=w43) -> ("Cursor.Cursor Position"=w45:T1)  [unwired: 1 in, 2 out]
            n58 = Unbundle By Name(w44) -> ("Cursor X"=w46:dbl, "Cursor Y"=w48:dbl)
            n59 = Unbundle By Name(w45) -> ("Cursor X"=w47:dbl, "Cursor Y"=w49:dbl)
            n60 = Max & Min(x=w46, y=w47) -> (max(x,y)=w50:dbl, min(x,y)=w51:dbl)
            n61 = Max & Min(x=w48, y=w49) -> (max(x,y)=w53:dbl, min(x,y)=w55:dbl)
            n62 = Index Array(array=w35, index (dim 0)="Current") -> (element=w37:i32[][][])  [unwired: 3 in]
            n63 = Subtract(x=w50, y=w51) -> (x-y=w52:dbl)
            n64 = Subtract(x=w53, y=w55) -> (x-y=w54:dbl)
            n65 = Array Subset(array=w37, index (dim 1)=w51, length (dim 1)=w52, index (dim 2)=w55, length (dim 2)=w54) -> (w41:i32[][][])  [unwired: 2 in]
            n66 = for {
              tunnel: [w57] -> w40 mode=indexing
              tunnel: w41 -> [w56] mode=indexing
              n67 = for {
                tunnel: w56 -> [w58] mode=indexing
                tunnel: [w58] -> w57 mode=concatenating
              }
            }
            n68 = Transpose 2D Array(2D array=w40) -> (transposed array=w34:i32[][])
            "ROI_Thscans" <- w34
          }
          frame #1 {
            # "Currents"
            n69 = To Single Precision Float(number=w65) -> (single precision float=w59:sgl[])
            n70 = property on="Image" class="IntGraph (strict)"("Active Cursor"=u32 1) -> (error out=w75:errorcluster)  [unwired: 2 in, 1 out]
            n71 = property on="Image" class="IntGraph (strict)"("Active Cursor"=u32 2) -> (error out=w76:errorcluster)  [unwired: 2 in, 1 out]
            n72 = property on="Image" class="IntGraph (strict)"(error in=w75) -> ("Cursor.Cursor Position"=w77:T1)  [unwired: 1 in, 2 out]
            n73 = property on="Image" class="IntGraph (strict)"(error in=w76) -> ("Cursor.Cursor Position"=w78:T1)  [unwired: 1 in, 2 out]
            n74 = Unbundle By Name(w77) -> ("Cursor X"=w79:dbl, "Cursor Y"=w81:dbl)
            n75 = Unbundle By Name(w78) -> ("Cursor X"=w80:dbl, "Cursor Y"=w82:dbl)
            n76 = Max & Min(x=w79, y=w80) -> (max(x,y)=w83:dbl, min(x,y)=w68:dbl)
            n77 = Max & Min(x=w81, y=w82) -> (max(x,y)=w84:dbl, min(x,y)=w70:dbl)
            n78 = Subtract(x=w83, y=w68) -> (x-y=w69:dbl)
            n79 = Subtract(x=w84, y=w70) -> (x-y=w71:dbl)
            n80 = property on="ROI_Thscans" class="WFGraph (strict)"() -> ("Cursor.Cursor Index"=w64:i32)  [unwired: 2 in, 2 out]
            n81 = Array Subset(array=w72, index (dim 2)=w68, length (dim 2)=w69, index (dim 3)=w70, length (dim 3)=w71) -> (w67:i32[][][][])  [unwired: 4 in]
            n82 = Index Array(array=w67, index (dim 1)=w64) -> (element=w66:i32[][][])  [unwired: 3 in]
            n83 = stacked-sequence {
              seq-local: [_ w102 _] -> [_ _ w137]
              tunnel: w66 -> [w87 w109 w146]
              tunnel: w59 -> [w86 w107 w138]
              tunnel: [w85 _ _] -> w62
              tunnel: [_ w116 _] -> w61
              tunnel: [_ _ w133] -> w60
              frame #0 {
                n84 = Index Array(array=w87, index (dim 0)=0 ("index (page)")) -> (element=w88:i32[][])  [unwired: 2 in]
                n85 = for {
                  tunnel: w88 -> [w94] mode=indexing
                  tunnel: w87 -> [w93]
                  tunnel: w86 -> [w91]
                  tunnel: [w90] -> w85 mode=concatenating
                  i -> [w92]
                  n86 = for {
                    tunnel: w94 -> [_] mode=indexing
                    tunnel: w93 -> [w101]
                    tunnel: w92 -> [w99]
                    tunnel: w91 -> [w97]
                    tunnel: [w95] -> w90 mode=indexing
                    i -> [w100]
                    n87 = Index Array(array=w101, index (dim 1)=w99, index (dim 2)=w100) -> (element=w96:i32[])  [unwired: 1 in]
                    n88 = Bundle By Name(cluster=cluster{"x":i32[], "y":i32[]} {"x"=[], "y"=[]}, "x"=w97, "y"=w96) -> (w95:cluster{"x":i32[], "y":i32[]})
                  }
                }
              }
              frame #1 {
                n89 = Index Array(array=w109, index (dim 0)=0 ("index (page)")) -> (element=w108:i32[][])  [unwired: 2 in]
                n90 = Multiply(x=w107, y=0 ("index (page)")) -> (x*y=w106:sgl[])
                n91 = for {
                  tunnel: w109 -> [w123]
                  shift-right: [w121] -> w111
                  shift-left: w106 -> [w122]
                  tunnel: [w120] -> w115
                  tunnel: [w119] -> w114
                  tunnel: w108 -> [w118] mode=indexing
                  i -> [w119]
                  n92 = for {
                    tunnel: w123 -> [w127]
                    shift-right: [w129] -> w121
                    shift-left: w122 -> [w128]
                    tunnel: [w124] -> w120
                    tunnel: w119 -> [w125]
                    tunnel: w118 -> [_] mode=indexing
                    i -> [w124]
                    n93 = Index Array(array=w127, index (dim 1)=w125, index (dim 2)=w124) -> (element=w126:i32[])  [unwired: 1 in]
                    n94 = Add(x=w128, y=w126) -> (x+y=w129:sgl[])
                  }
                }
                n95 = Increment(x=w115) -> (x+1=w104:i32)
                n96 = Increment(x=w114) -> (x+1=w103:i32)
                n97 = Multiply(x=w104, y=w103) -> (x*y=w113:i32)
                n98 = Divide(x=w111, y=w113) -> (x/y=w112:sgl[])
                n99 = To Long Integer(number=w112) -> (32bit integer=w102:i32[])
                n100 = Bundle By Name(cluster=cluster{"x":i32[], "y":i32[]} {"x"=[], "y"=[]}, "x"=w107, "y"=w102) -> (w116:cluster{"x":i32[], "y":i32[]})
              }
              frame #2 {
                w139 = cluster{"x":i32[], "y":i32[]} {"x"=[], "y"=[]}
                n101 = Index Array(array=w146, index (dim 0)=0 ("index (page)")) -> (element=w145:i32[][])  [unwired: 2 in]
                n102 = Multiply(x=w138, y=0 ("index (page)")) -> (x*y=w144:sgl[])
                n103 = for {
                  tunnel: w146 -> [w158]
                  shift-right: [w156] -> w148
                  shift-left: w144 -> [w157]
                  tunnel: [w155] -> w151
                  tunnel: [w154] -> w150
                  tunnel: w145 -> [w153] mode=indexing
                  tunnel: w137 -> [w152]
                  i -> [w154]
                  n104 = for {
                    tunnel: w158 -> [w165]
                    shift-right: [w167] -> w156
                    shift-left: w157 -> [w166]
                    tunnel: [w163] -> w155
                    tunnel: w154 -> [w164]
                    tunnel: w153 -> [_] mode=indexing
                    tunnel: w152 -> [w162]
                    i -> [w163]
                    n105 = Index Array(array=w165, index (dim 1)=w164, index (dim 2)=w163) -> (element=w161:i32[])  [unwired: 1 in]
                    n106 = Subtract(x=w162, y=w161) -> (x-y=w160:i32[])
                    n107 = Square(x=w160) -> (x^2=w159:i32[])
                    n108 = Add(x=w166, y=w159) -> (x+y=w167:sgl[])
                  }
                }
                n109 = Increment(x=w151) -> (x+1=w142:i32)
                n110 = Increment(x=w150) -> (x+1=w141:i32)
                n111 = Multiply(x=w142, y=w141) -> (x*y=w149:i32)
                n112 = Divide(x=w148, y=w149) -> (x/y=w131:sgl[])
                n113 = Square Root(x=w131) -> (sqrt(x)=w130:sgl[])
                n114 = To Long Integer(number=w130) -> (32bit integer=w136:i32[])
                n115 = Subtract(x=w137, y=w136) -> (x-y=w135:i32[])
                n116 = Add(x=w137, y=w136) -> (x+y=w140:i32[])
                n117 = Bundle By Name(cluster=w139, "x"=w138, "y"=w135) -> (w134:cluster{"x":i32[], "y":i32[]})
                n118 = Bundle By Name(cluster=w139, "x"=w138, "y"=w140) -> (w132:cluster{"x":i32[], "y":i32[]})
                n119 = Build Array(w134, w132) -> (w133:cluster{"x":i32[], "y":i32[]}[])
              }
            }
            n120 = Build Array (concatenate)(w61, w60, w62) -> (→"ROI Counns_vs_Current":cluster{"x":i32[], "y":i32[]}[])
          }
        }
      }
      frame #2 {
        # "Image"
        n121 = local read "Current"() -> (w170:u16)
        n122 = property on="SP_Thscans" class="WFGraph (strict)"() -> ("Cursor.Cursor Index"=w172:i32)  [unwired: 2 in, 2 out]
        n123 = Index Array(array=w168, index (dim 0)=w170) -> (element=w169:i32[][][])  [unwired: 3 in]
        n124 = Index Array(array=w169, index (dim 0)=w172) -> (element=→"Image":i32[][])  [unwired: 2 in]
      }
      frame #3 {
      }
    }
  }
